vi "One-PID.vi"(7 "Reset":bool, 8 "Error In":errorcluster, 11 "目標角度":dbl) -> (0 "Error Out":errorcluster)   [LabVIEW 2019]
uses:
  <vilib>/addons/control/pid/pid.llb/PID (DBL).vi
  <vilib>/addons/control/pid/NI_PID_pid.lvlib
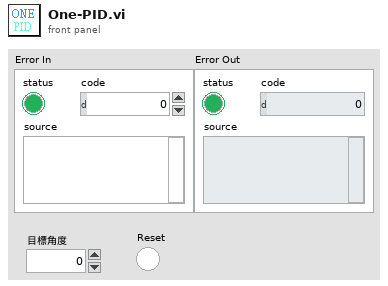
[diagram p1: front panel]
types:
  T1 = cluster{"proportional gain (Kc)":dbl, "integral time (Ti, min)":dbl, "derivative time (Td, min)":dbl}
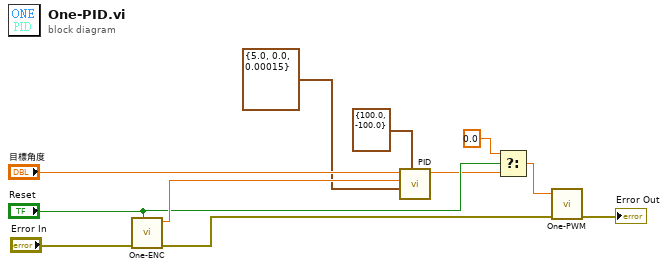
[diagram p0: block diagram]
diagram:
  n1 = call "One-ENC.vi"("Reset"="Reset", "Error In"="Error In") -> ("Error Out"=w9:errorcluster, "Counter Value"=w8:dbl)  [unwired: 8 in]
  n2 = call-poly <vilib>:"PID.vi"("output range"=cluster{"output high":dbl, "output low":dbl} {"output high"=100.0, "output low"=-100.0}, "PID gains"=T1 {"proportional gain (Kc)"=5.0, "integral time (Ti, min)"=0.0, "derivative time (Td, min)"=0.00015}, "process variable"=w8, "setpoint"="目標角度") -> ("output"=w3:dbl)  [unwired: 6 in, 1 out]
  n3 = Select(t=0.0, s="Reset", f=w3) -> (s? t:f=w4:dbl)
  n4 = call "One-PWM.vi"("Error In"=w9, "Duty Cycle"=w4) -> ("Error Out"=→"Error Out":errorcluster)  [unwired: 9 in]
